vi "running_as_admin.vi"(8 "error in (no error)":errorcluster) -> (0 "error out":errorcluster, 3 "admin":bool)   [LabVIEW 2015, in "lv-bin-windows.lvlib" / "v1.lvlib"]
uses:
  v1.lvlib
  <userlib>/antonio-alexander/lv-bin/lv-bin/public/api/v1/v1.lvlib
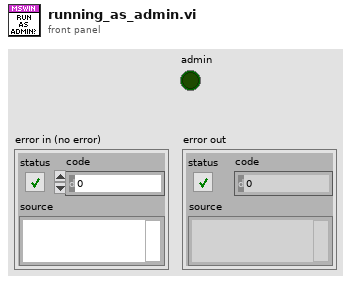
[diagram p1: front panel]
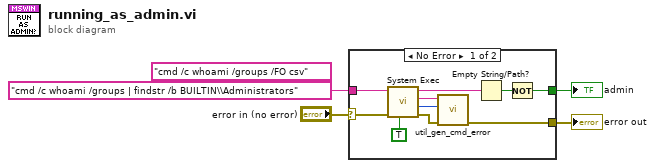
[diagram p0: block diagram]
diagram:
  (unwired) "cmd /c whoami /groups /FO csv"
  n1 = case shown="No Error" "error in (no error)" {
    selector: "error in (no error)" -> [w14 w15]
    tunnel: "cmd /c whoami /groups | findstr /b BUILTIN\\Administrators" -> [w9 _]
    tunnel: [w8 w15] -> w2
    tunnel: [w5 _] -> w1
    frame No Error {
      n2 = call <vilib>:"System Exec.vi"("run minimized? (F)"=TRUE, "error in (no error)"=w14, "command line"=w9) -> ("error out"=w12:errorcluster, "return code"=w10:i32, "standard error"=w11:string, "standard output"=w7:string)  [unwired: 5 in]
      n3 = call <userlib>:"util_gen_cmd_error.vi"("error in (no error)"=w12, "return_code"=w10, "standard_error"=w11) -> ("error out"=w8:errorcluster)  [unwired: 8 in]
      n4 = Empty String/Path?(string/path=w7) -> (empty?=w6:bool)
      n5 = Not(x=w6) -> (.not. x?=w5:bool)
    }
    frame Error {
    }
  }
  "admin" <- w1
  "error out" <- w2
